vi "FlyWheelCtrl_Example.vi"() -> ()   [LabVIEW 2019]
uses:
  <vilib>/Rock Robotics/WPI/ThirdParty/JAS_Junk/TrajLib/TypeDef/DCMOTOR.CTL
  <vilib>/Rock Robotics/WPI/ThirdParty/JAS_Junk/TrajLib/TypeDef/LINEAR_SYSTEM.ctl
  <vilib>/Analysis/Matrix/Datatypes/RealMatrix.ctl
  <vilib>/Rock Robotics/WPI/ThirdParty/JAS_Junk/TrajLib/TypeDef/FLYWHEEL_SIM.ctl
  <vilib>/Rock Robotics/WPI/ThirdParty/JAS_Junk/TrajLib/TypeDef/LINEAR_SYSTEM_SIM.ctl
  <vilib>/Rock Robotics/WPI/ThirdParty/JAS_Junk/TrajLib/Enum/DCMOTOR_TYPES_ENUM.ctl
  <vilib>/Rock Robotics/WPI/ThirdParty/JAS_Junk/TrajLib/VI/BoolCmd_Send_Internal.vi
  <vilib>/Rock Robotics/WPI/ThirdParty/JAS_Junk/TrajLib/VI/numCmd_ObtainQueue_OneDbl.vi
  <vilib>/Rock Robotics/WPI/ThirdParty/JAS_Junk/TrajLib/VI/BoolCmd_Recv_Internal.vi
  <vilib>/Rock Robotics/WPI/ThirdParty/JAS_Junk/TrajLib/LinearFilter_ResetToValue.vi
  <vilib>/Rock Robotics/WPI/ThirdParty/JAS_Junk/TrajLib/LinearFilter_Calculate.vi
  <vilib>/Rock Robotics/WPI/ThirdParty/JAS_Junk/TrajLib/VI/BoolCmd_ObtainQueue.vi
  <vilib>/Rock Robotics/WPI/ThirdParty/JAS_Junk/TrajLib/LinearFilter_MovingAverage.vi
  <vilib>/Rock Robotics/WPI/ThirdParty/JAS_Junk/TrajLib/LinearFilter_LowPassBW1.vi
  <vilib>/Rock Robotics/WPI/ThirdParty/JAS_Junk/TrajLib/LinearFilter_LowPassBW2.vi
  <vilib>/Rock Robotics/WPI/ThirdParty/JAS_Junk/TrajLib/LinearFilter_HighPassBW1.vi
  <vilib>/Rock Robotics/WPI/ThirdParty/JAS_Junk/TrajLib/LinearFilter_HighPassBW2.vi
  <vilib>/Rock Robotics/WPI/ThirdParty/JAS_Junk/TrajLib/Trajectory_Library.lvlib
  <vilib>/Analysis/Matrix/NI_Matrix.lvlib
panel:
  in  "Tab Control":T1(tab)
  in  "Speed Setpoint RPM":dbl=2500.0 format="%20.3f"
  out "Motor Current":dbl format="%20.3f"
  out "Battery \nVoltage":dbl format="%20.3f"
  in  "Shoot ball":bool
  out "CO Chart":T2(graph)
  in  "Shooter On/Off":bool
  out "Encoer Speed\nRPM":dbl(slide) scale=0.0..5500.0
  out "Speed RPM":dbl format="%20.3f"
  out "Kalman Filtered\nSpeed RPM":dbl format="%20.3f"
  out "PV Chart":T3(graph)
  out "Controller Error":bool
  out "Motor Volt Dmd (CO)":dbl format="%20.3f"
  out "shoot Start":bool
  out "Shoot Done":bool
  out "Shooter Motor":T4 {"Jr_KgM2" format="%13.5p"; "L_H" format="%13.5p"; "Kt_NMPerAmp" format="%13.5p"; "KvINV_RadPerSecPerVolt" format="%13.5p"; "R_Ohms" format="%13.5p"; "FreeSpeed_RadPerSec" format="%13.5p"; "FreeCurrent_Amps" format="%13.5p"; "StallCurrent_Amps" format="%13.5p"; "StallTorque_NM" format="%13.5p"; "nominalVoltage_Volts" format="%13.5p"}
  out "m_flywheelPlant":T5
  out "m_FlyWheelSim":T7 {"GearBox"."Jr_KgM2" format="%13.5p"; "GearBox"."L_H" format="%13.5p"; "GearBox"."Kt_NMPerAmp" format="%13.5p"; "GearBox"."KvINV_RadPerSecPerVolt" format="%13.5p"; "GearBox"."R_Ohms" format="%13.5p"; "GearBox"."FreeSpeed_RadPerSec" format="%13.5p"; "GearBox"."FreeCurrent_Amps" format="%13.5p"; "GearBox"."StallCurrent_Amps" format="%13.5p"; "GearBox"."StallTorque_NM" format="%13.5p"; "GearBox"."nominalVoltage_Volts" format="%13.5p"}
  out "Shooting A":T6
  out "Shooting B":T6
  # "<States,States>"
  # "<States,Inputs>"
  # "<Outputs,States>"
  # "<Outputs,Inputs>"
  # "<States, 1>"
  # "<Outputs, 1>"
  # "<Inputs, 1>"
  # "<Outputs, 1>"
  # "<States,States>"
  # "<States,Inputs>"
  # "<Outputs,States>"
  # "<Outputs,Inputs>"
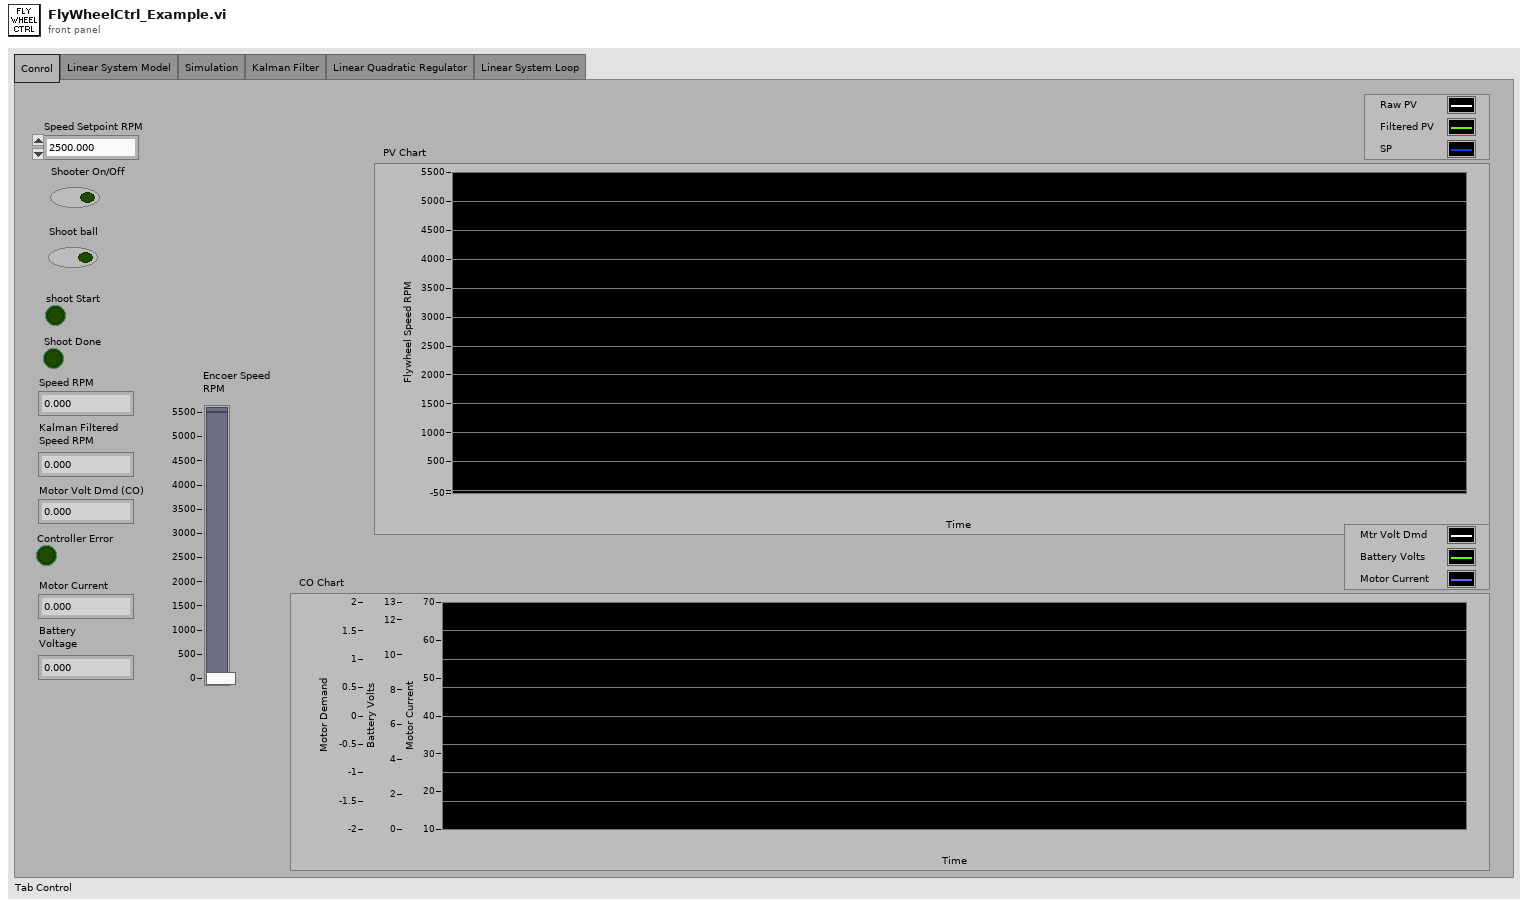
[diagram p1: front panel]
types:
  T1 = enum32{"Conrol", "Linear System Model", "Simulation", "Kalman Filter", "Linear Quadratic Regulator", "Linear System Loop"}
  T2 = cluster{"f":dbl, "Voltage":dbl, "Motor Current":dbl}
  T3 = cluster{"upper limit":dbl, "Real Matrix Element":dbl, "Real Matrix Element":dbl}
  T4 = typedef "Trajectory_Library.lvlib/DCMOTOR.CTL" = cluster{"nominalVoltage_Volts":dbl, "StallTorque_NM":dbl, "StallCurrent_Amps":dbl, "FreeCurrent_Amps":dbl, "FreeSpeed_RadPerSec":dbl, "R_Ohms":dbl, "KvINV_RadPerSecPerVolt":dbl, "Kt_NMPerAmp":dbl, "L_H":dbl, "Jr_KgM2":dbl}
  T5 = typedef "Trajectory_Library.lvlib/LINEAR_SYSTEM.ctl" = cluster{"m_A":T6, "m_B":T6, "m_C":T6, "m_D":T6, "States":i32, "Inputs":i32, "Outputs":i32}
  T6 = typedef "NI_Matrix.lvlib/RealMatrix.ctl" = dbl[][]
  T7 = typedef "Trajectory_Library.lvlib/FLYWHEEL_SIM.ctl" = cluster{"LinearSystemSim":T8, "GearBox":T4, "Gearing":dbl}
  T8 = typedef "Trajectory_Library.lvlib/LINEAR_SYSTEM_SIM.ctl" = cluster{"m_Plant":T5, "m_X":T6, "m_Y":T6, "m_U":T6, "MeasureStdDev":T6}
  T9 = enum16{"Moving Average", "Low Pass 1st Order Butterworth", "Low Pass 2nd Order Butterworth", "High Pass 1st Order Butterworth", "High Pass 2nd Order Butterworth"}
  T10 = cluster{"RotationsPerMinute":dbl, "Value":dbl, "Value":dbl}
  T11 = typedef "Trajectory_Library.lvlib/DCMOTOR_TYPES_ENUM.ctl" = enum16{"CIM", "AndyMark 9015", "Andy Mark RS 775 125", "Bag", "BaneBots RS 550", "BaneBots RS 775", "Falcon 500", "Mini CIM", "NEO", "NEO 550", "Romi BuiltIn", "Vex 775 Pro", "Snow Blower AM 2235A", "Bosch Seat AM 3493"}
  T12 = typedef "Trajectory_Library.lvlib/LINEAR_SYSTEM_ID_FLYWHEEL_MODEL.ctl" = cluster{"DCMOTOR_TYPES":T11, "Num Motors":i32, "Gearing":dbl, "MOI kgm2":dbl}
  T13 = typedef "Trajectory_Library.lvlib/LINEAR_SYSTEM_LOOP_FLYWHEEL_CTRL_PARAMS.CTL" = cluster{"Vel Model Std Dev Rad/Sec":dbl, "Vel Meas Std Dev Rad/Sec":dbl, "Vel Ctrl Tol Rad/Sec":dbl, "Max Ctrl Out V":dbl}
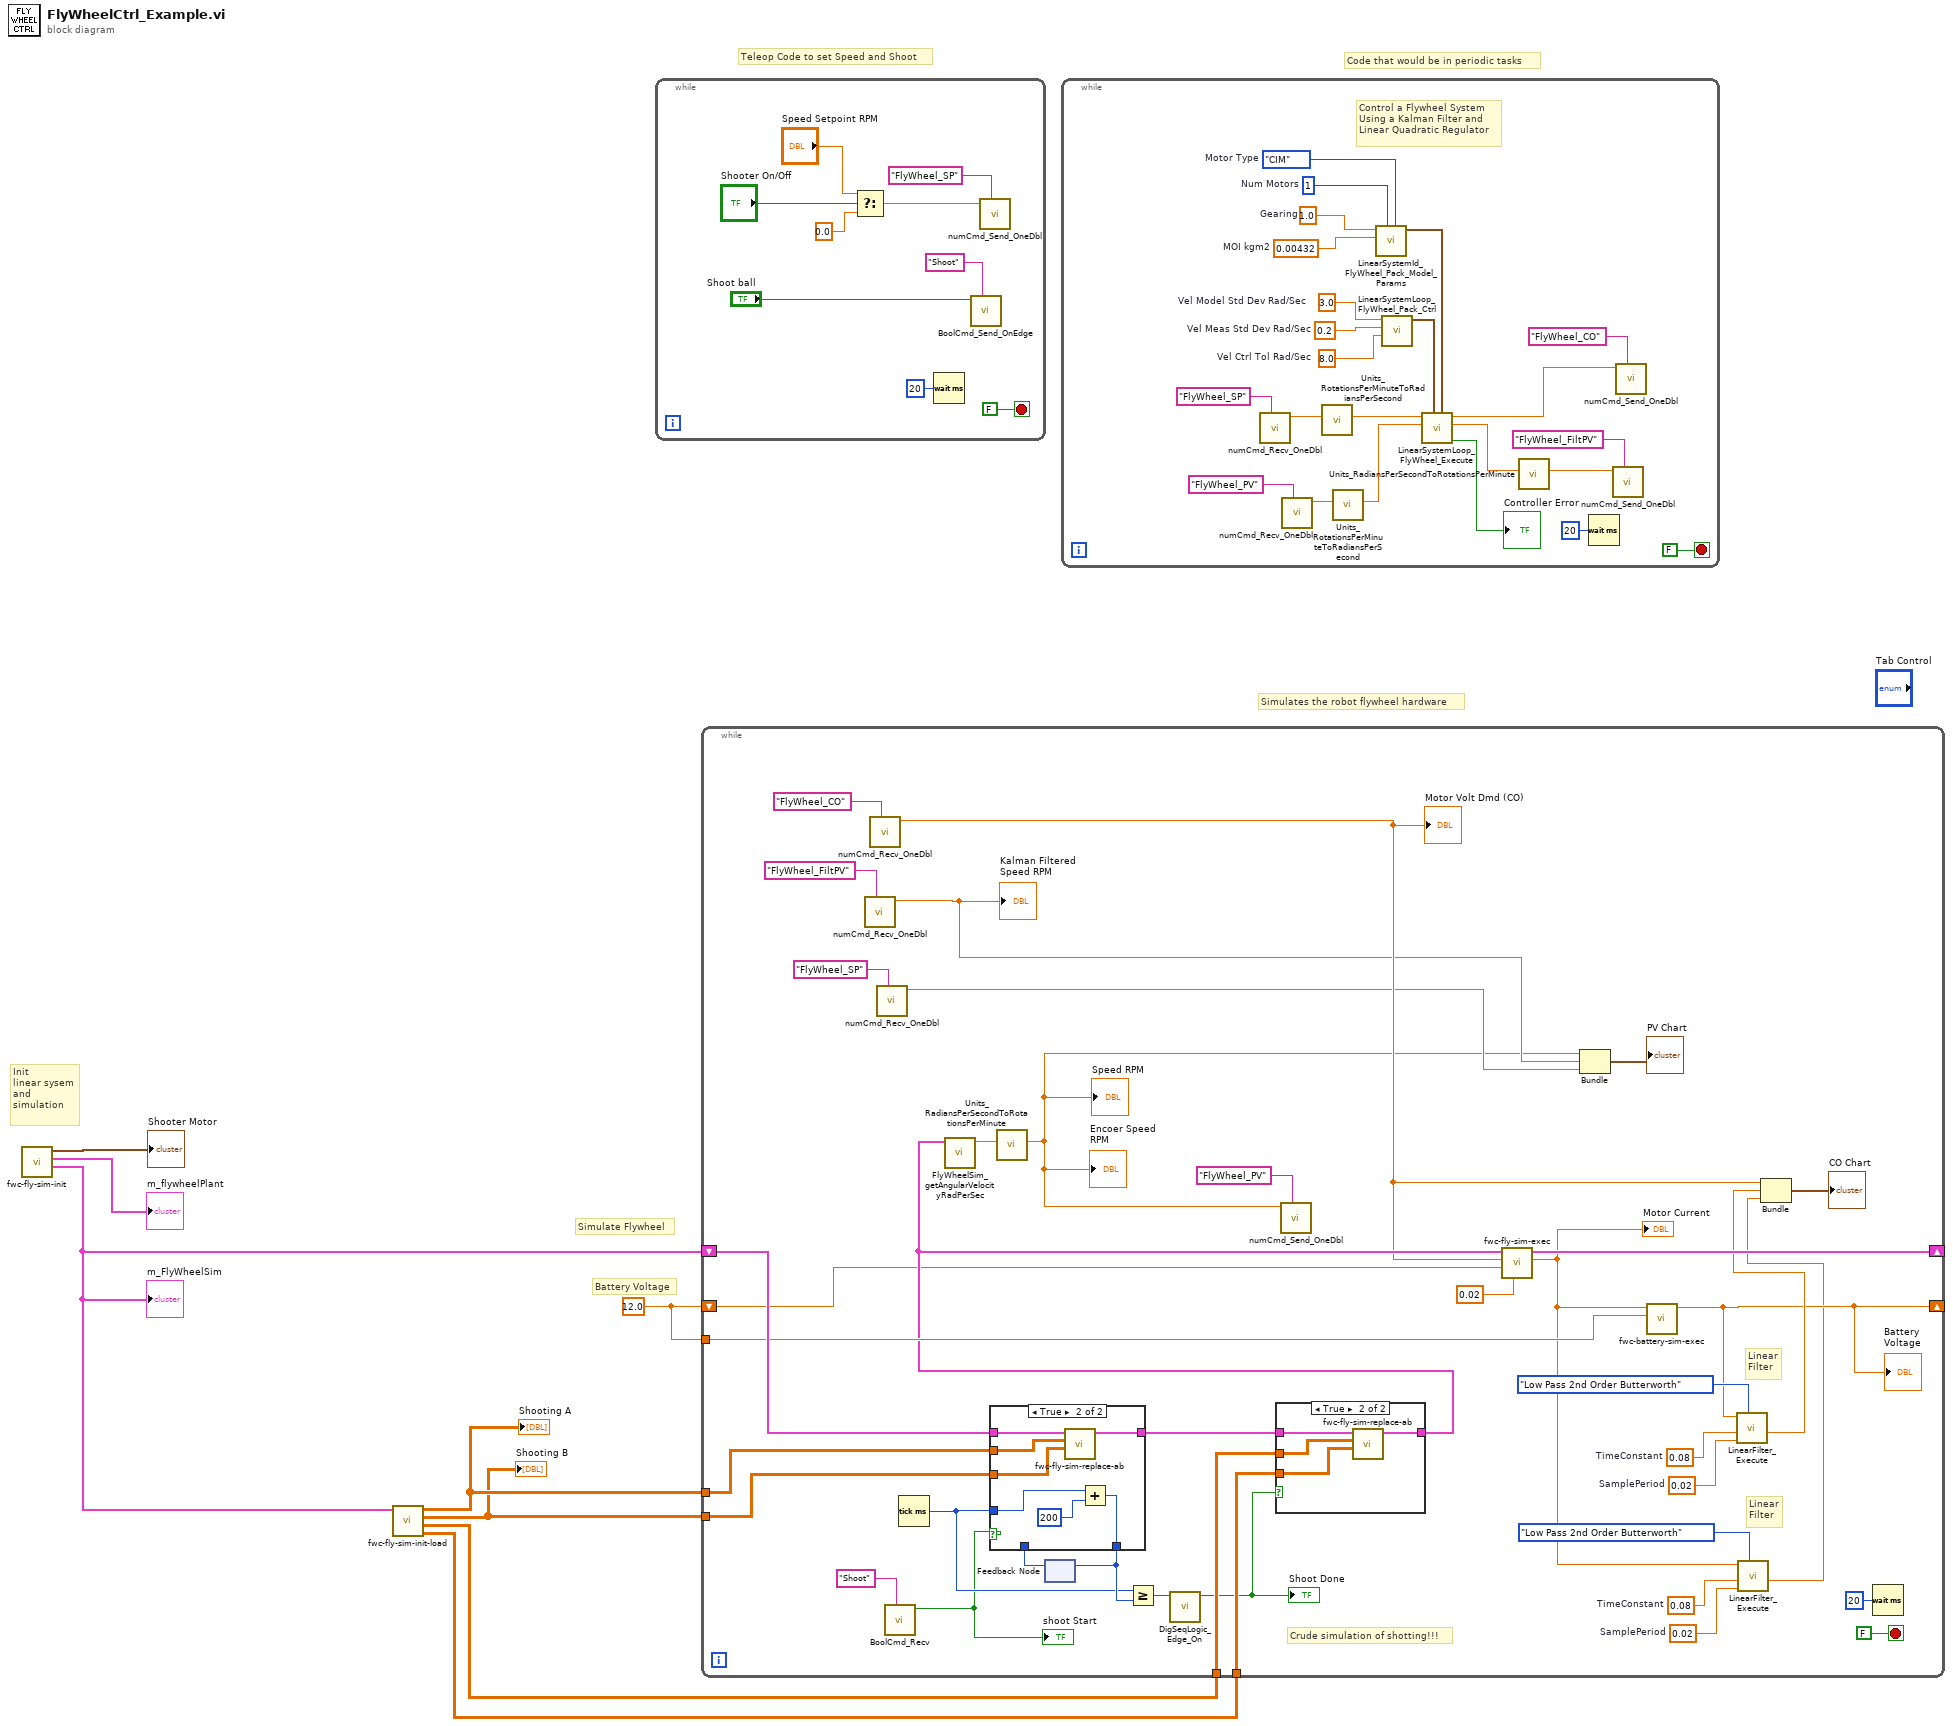
[diagram p0: block diagram]
diagram:
  w7 = 12.0
  # "Teleop Code to set Speed and Shoot"
  # "Code that would be in periodic tasks"
  # "Simulates the robot flywheel hardware"
  # "Init\nlinear sysem\nand \nsimulation"
  # "Simulate Flywheel"
  # "Battery Voltage"
  n1 = call "fwc-fly-sim-init.vi"() -> ("FlyWheelSim"=w6:T7, "Linearsystem"=→"m_flywheelPlant":T5, "DCMOTOR"=→"Shooter Motor":T4)  [unwired: 9 in]
  "m_FlyWheelSim" <- w6
  n2 = call "fwc-fly-sim-init-load.vi"("FlyWheelSim"=w6) -> ("Normal B"=w1:T6, "Normal A"=w2:T6, "Loaded B"=w4:T6, "Loaded A"=w5:T6)  [unwired: 7 in]
  "Shooting A" <- w5
  "Shooting B" <- w4
  n3 = while {
    stop <- FALSE stop-if-true
    n4 = Select(t="Speed Setpoint RPM", s="Shooter On/Off", f=0.0) -> (s? t:f=w14:dbl)
    n5 = Wait (ms)(milliseconds to wait=u32 20) -> ()  [unwired: 1 out]
    n6 = call <vilib>:"BoolCmd_Send_OnEdge.vi"("Command Name"="Shoot", "Value"="Shoot ball") -> ()  [unwired: 9 in, 1 out]
    n7 = call <vilib>:"numCmd_Send_OneDbl.vi"("Command Name"="FlyWheel_SP", "Value"=w14) -> ()  [unwired: 9 in, 1 out]
  }
  n8 = while {
    shift-right: [w55] -> _
    shift-left: w6 -> [w53]
    shift-right: [w33] -> _
    shift-left: w7 -> [w41]
    tunnel: w7 -> [w45]
    tunnel: w2 -> [w51]
    tunnel: w1 -> [w50]
    tunnel: w5 -> [w49]
    tunnel: w4 -> [w48]
    stop <- FALSE stop-if-true
    w37 = 0.02  # SamplePeriod
    w36 = 0.08  # TimeConstant
    w40 = 0.02  # SamplePeriod
    w39 = 0.08  # TimeConstant
    # "Linear\nFilter"
    # "Linear\nFilter"
    # "Crude simulation of shotting!!!"
    n9 = call <vilib>:"numCmd_Recv_OneDbl.vi"("Command Name"="FlyWheel_FiltPV") -> ("Value"=w27:dbl)  [unwired: 8 in, 2 out]
    "Kalman Filtered\nSpeed RPM" <- w27
    n10 = call <vilib>:"numCmd_Recv_OneDbl.vi"("Command Name"="FlyWheel_CO") -> ("Value"=w29:dbl)  [unwired: 8 in, 2 out]
    "Motor Volt Dmd (CO)" <- w29
    n11 = call <vilib>:"numCmd_Recv_OneDbl.vi"("Command Name"="FlyWheel_SP") -> ("Value"=w25:dbl)  [unwired: 8 in, 2 out]
    n12 = call <vilib>:"BoolCmd_Recv.vi"("Command Name"="Shoot") -> ("New Request"=w18:bool)  [unwired: 9 in, 1 out]
    "shoot Start" <- w18
    n13 = Tick Count (ms)() -> (millisecond timer value=w44:u32)
    n14 = feedback #1() -> (w46:u32)  [unwired: 1 in]
    n15 = case shown="True" w18 {
      tunnel: w53 -> [w65 w70]
      tunnel: [w65 w69] -> w52
      tunnel: w49 -> [_ w68]
      tunnel: w48 -> [_ w67]
      tunnel: [w64 w71] -> w47
      tunnel: w46 -> [w64 _]
      tunnel: w44 -> [_ w66]
      frame False {
      }
      frame True {
        n16 = call "fwc-fly-sim-replace-ab.vi"("B"=w67, "A"=w68, "in FlyWheelSim"=w70) -> ("out FlyWheelSim"=w69:T7)  [unwired: 8 in]
        n17 = Add(x=w66, y=u32 200) -> (x+y=w71:u32)
      }
    }
    n18 = feedback-in #1(w47) -> ()
    n19 = Greater Or Equal?(x=w44, y=w47) -> (x >= y?=w20:bool)
    n20 = call <vilib>:"DigSeqLogic_Edge_On.vi"("Input"=w20) -> ("On Edge"=w21:bool)  [unwired: 10 in]
    "Shoot Done" <- w21
    n21 = case shown="True" w21 {
      tunnel: w52 -> [w59 w63]
      tunnel: [w59 w62] -> w42
      tunnel: w51 -> [_ w61]
      tunnel: w50 -> [_ w60]
      frame False {
      }
      frame True {
        n22 = call "fwc-fly-sim-replace-ab.vi"("B"=w60, "A"=w61, "in FlyWheelSim"=w63) -> ("out FlyWheelSim"=w62:T7)  [unwired: 8 in]
      }
    }
    n23 = call <vilib>:"FlyWheelSim_getAngularVelocityRadPerSec.vi"("FlyWheelSim"=w42) -> ("Velocity_RadPerSec"=w24:dbl)  [unwired: 10 in]
    n24 = call <vilib>:"Units_RadiansPerSecondToRotationsPerMinute.vi"("RadiansPerSecond"=w24) -> ("RotationsPerMinute"=w22:dbl)  [unwired: 10 in]
    "Encoer Speed\nRPM" <- w22
    "Speed RPM" <- w22
    n25 = call <vilib>:"numCmd_Send_OneDbl.vi"("Command Name"="FlyWheel_PV", "Value"=w22) -> ()  [unwired: 9 in, 1 out]
    n26 = call "fwc-fly-sim-exec.vi"("dT_Seconds"=0.02, "Battery Voltage"=w41, "Motor Dmd (CO)"=w29, "in FlyWheelSim"=w42) -> ("Motor Current"=w32:dbl, "out FlyWheelSim"=w55:T7)  [unwired: 6 in]
    "Motor Current" <- w32
    n27 = Bundle("RotationsPerMinute"=w22, "Value"=w27, "Value"=w25) -> (→"PV Chart":T10)  [unwired: 1 in]
    n28 = call "fwc-battery-sim-exec.vi"("Numeric"=w45, "Motor Current"=w32) -> ("Voltage"=w33:dbl)  [unwired: 9 in]
    "Battery \nVoltage" <- w33
    n29 = call <vilib>:"LinearFilter_Execute.vi"("Filter Type"=T9."Low Pass 2nd Order Butterworth", "SamplePeriod"=w40, "TimeConstant"=w39, "Input"=w33) -> ("Output"=w34:dbl)  [unwired: 6 in, 1 out]
    n30 = call <vilib>:"LinearFilter_Execute.vi"("Filter Type"=T9."Low Pass 2nd Order Butterworth", "SamplePeriod"=w37, "TimeConstant"=w36, "Input"=w32) -> ("Output"=w31:dbl)  [unwired: 6 in, 1 out]
    n31 = Bundle("Value"=w29, "Output"=w34, "Output"=w31) -> (→"CO Chart":cluster{"Value":dbl, "Output":dbl, "Output":dbl})  [unwired: 1 in]
    n32 = Wait (ms)(milliseconds to wait=u32 20) -> ()  [unwired: 1 out]
  }
  n33 = while {
    stop <- FALSE stop-if-true
    w85 = 3.0  # Vel Model Std Dev Rad/Sec
    w86 = 0.2  # Vel Meas Std Dev Rad/Sec
    w87 = 8.0  # Vel Ctrl Tol Rad/Sec
    w92 = 1.0  # Gearing
    w93 = 0.00432  # MOI kgm2
    w94 = 1  # Num Motors
    w95 = DCMOTOR_TYPES_ENUM."CIM"  # Motor Type
    # "Control a Flywheel System\nUsing a Kalman Filter and \nLinear Quadratic Regulator"
    n34 = call <vilib>:"numCmd_Recv_OneDbl.vi"("Command Name"="FlyWheel_SP") -> ("Value"=w79:dbl)  [unwired: 8 in, 2 out]
    n35 = call <vilib>:"numCmd_Recv_OneDbl.vi"("Command Name"="FlyWheel_PV") -> ("Value"=w83:dbl)  [unwired: 8 in, 2 out]
    n36 = call <vilib>:"Units_RotationsPerMinuteToRadiansPerSecond.vi"("RotationsPerMinute"=w79) -> ("RadiansPerSecond"=w81:dbl)  [unwired: 10 in]
    n37 = call <vilib>:"Units_RotationsPerMinuteToRadiansPerSecond.vi"("RotationsPerMinute"=w83) -> ("RadiansPerSecond"=w82:dbl)  [unwired: 10 in]
    n38 = call <vilib>:"LinearSystemId_FlyWheel_Pack_Model_Params.vi"("DCMOTOR_TYPES"=w95, "Num Motors"=w94, "MOI kgm2"=w93, "Gearing"=w92) -> ("LinearSystem_ID_FlyWheel_Model"=w89:T12)  [unwired: 7 in]
    n39 = call <vilib>:"LinearSystemLoop_FlyWheel_Pack_Ctrl.vi"("Vel Ctrl Tol Rad/Sec"=w87, "Vel Meas Std Dev Rad/Sec"=w86, "Vel Model Std Dev Rad/Sec"=w85) -> ("LinearSystemLoop_FlyWheel_Ctrl_Params"=w88:T13)  [unwired: 8 in]
    n40 = call <vilib>:"LinearSystemLoop_FlyWheel_Execute.vi"("FlyWheelSim_Model _Params"=w89, "LinearSystem_FlyWheel_Ctrl_Params"=w88, "Velocity (Rad/Sec)\n(PV)"=w82, "Velocity (Rad/Sec)\nSetpoint (SP)"=w81) -> ("Error"=→"Controller Error":bool, "Kalman FIltered\nVelocity (PV)"=w74:dbl, "Motor Dmd"=w77:dbl)  [unwired: 5 in]
    n41 = call <vilib>:"Units_RadiansPerSecondToRotationsPerMinute.vi"("RadiansPerSecond"=w74) -> ("RotationsPerMinute"=w75:dbl)  [unwired: 10 in]
    n42 = Wait (ms)(milliseconds to wait=u32 20) -> ()  [unwired: 1 out]
    n43 = call <vilib>:"numCmd_Send_OneDbl.vi"("Command Name"="FlyWheel_FiltPV", "Value"=w75) -> ()  [unwired: 9 in, 1 out]
    n44 = call <vilib>:"numCmd_Send_OneDbl.vi"("Command Name"="FlyWheel_CO", "Value"=w77) -> ()  [unwired: 9 in, 1 out]
  }
